vi "Add Rock Lines to Grid.vi"(8 "Rock Lines":cluster{"Array":u32[][]}[](array[cluster]), 9 "Column Offset":i32, 11 "Grig in":T1[][](array[typedef])) -> (3 "Grig out":T1[][](array[typedef]))   [LabVIEW 2020]
uses:
  RB ENUM_Space ID.ctl
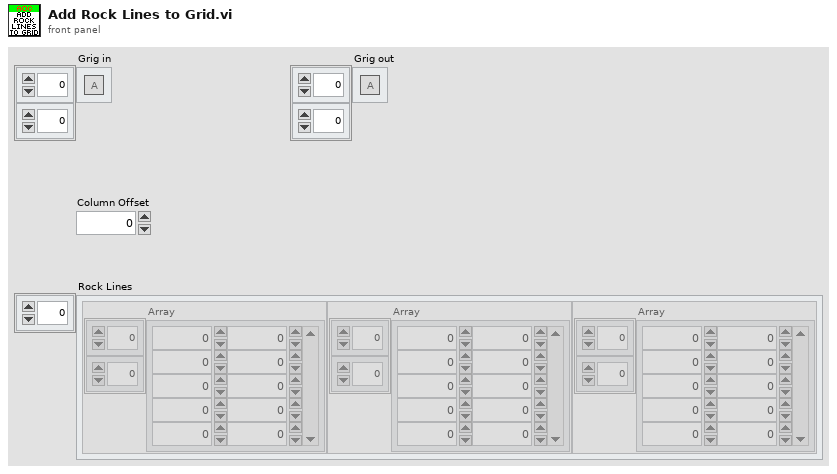
[diagram p1: front panel]
types:
  T1 = typedef "RB ENUM_Space ID.ctl" = enum32{"Air", "Sand", "Rock", "Start", "Abyss"}
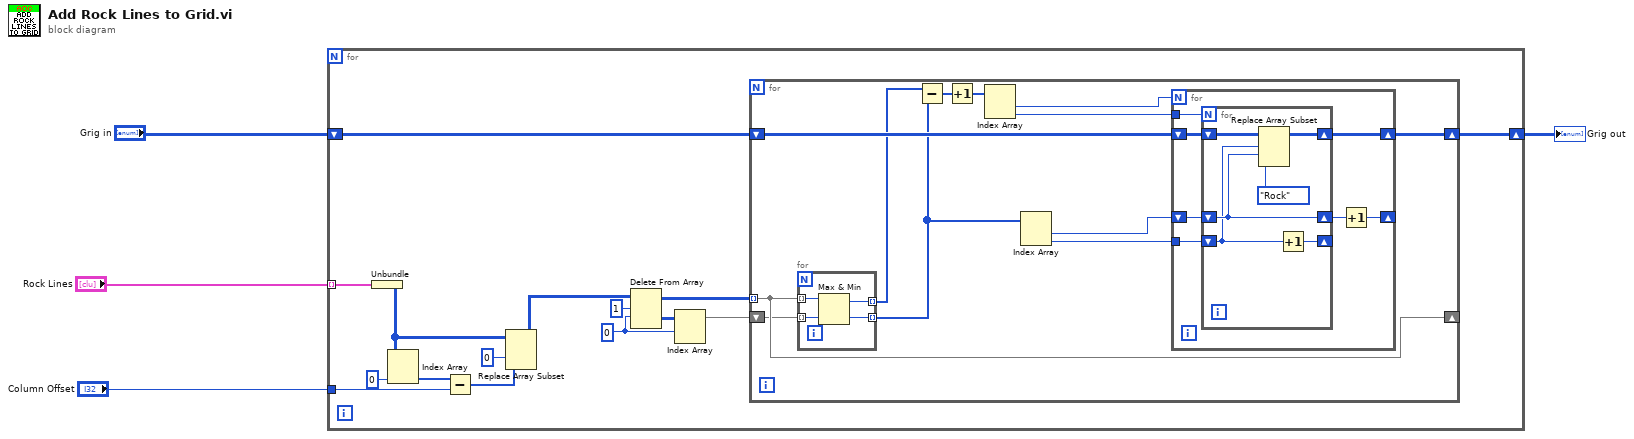
[diagram p0: block diagram]
diagram:
  n1 = for {
    shift-right: [w15] -> w2
    shift-left: "Grig in" -> [w16]
    tunnel: "Rock Lines" -> [w19] mode=indexing
    tunnel: "Column Offset" -> [w9]
    w12 = 0 ("index (row)")
    n2 = Unbundle(w19) -> ("Array"=w7:u32[][])
    n3 = Index Array(array=w7, index (col)=0 ("disabled index (col)")) -> (element=w10:u32[])  [unwired: 1 in]
    n4 = Subtract(x=w10, y=w9) -> (x-y=w8:u32[])
    n5 = Replace Array Subset(array=w7, new element=w8, index (col)=0 ("disabled index (col)")) -> (w5:u32[][])  [unwired: 1 in]
    n6 = Delete From Array(array=w5, length=1 ("index (row)"), index (row)=w12) -> (deleted portion=w14:u32[][], array with subset deleted=w17:u32[][])  [unwired: 1 in]
    n7 = Index Array(array=w14, index (row)=w12) -> (element=w13:u32[])  [unwired: 1 in]
    n8 = for {
      tunnel: w17 -> [w23] mode=indexing
      shift-right: [w23] -> _
      shift-left: w13 -> [w22]
      shift-right: [w29] -> w15
      shift-left: w16 -> [w30]
      n9 = for {
        tunnel: w23 -> [w34] mode=indexing
        tunnel: w22 -> [w35] mode=indexing
        tunnel: [w33] -> w21 mode=indexing
        tunnel: [w32] -> w20 mode=indexing
        n10 = Max & Min(x=w34, y=w35) -> (max(x,y)=w33:u32, min(x,y)=w32:u32)
      }
      n11 = Subtract(x=w21, y=w20) -> (x-y=w31:u32[])
      n12 = Increment(x=w31) -> (x+1=w26:u32[])
      n13 = Index Array(array=w26) -> (element #1=w28:u32, element #2=w27:u32)  [unwired: 2 in]
      n14 = Index Array(array=w20) -> (element #1=w24:u32, element #2=w25:u32)  [unwired: 2 in]
      n15 = for {
        N: w28 -> [_]
        shift-right: [w41] -> w29
        shift-left: w30 -> [w42]
        tunnel: w27 -> [w40]
        tunnel: w25 -> [w39]
        shift-right: [w36] -> _
        shift-left: w24 -> [w38]
        n16 = for {
          N: w40 -> [_]
          shift-right: [w46] -> w41
          shift-left: w42 -> [w47]
          shift-right: [w48] -> _
          shift-left: w39 -> [w43]
          shift-right: [w44] -> w37
          shift-left: w38 -> [w44]
          n17 = Replace Array Subset(array=w47, new element=RB_ENUM_Space_ID."Rock" ("Space"), index (row)=w43, index (col)=w44) -> (w46:T1[][])
          n18 = Increment(x=w43) -> (x+1=w48:u32)
        }
        n19 = Increment(x=w37) -> (x+1=w36:u32)
      }
    }
  }
  "Grig out" <- w2
